vi "Test Gamma jj'.vi"() -> ()   [LabVIEW 2013, in "Zernike Polynome.lvlib"]
doc: "This VI is used to test the calculation of the Zernike polynomial derivative matrix."
uses:
  Zernike Polynome.lvlib
panel:
  out "Array 2":dbl[][](array[numeric])
  out "Array":T1(array[cluster])
  in  "X/Y":bool
  in  "j max (1)":i32=1
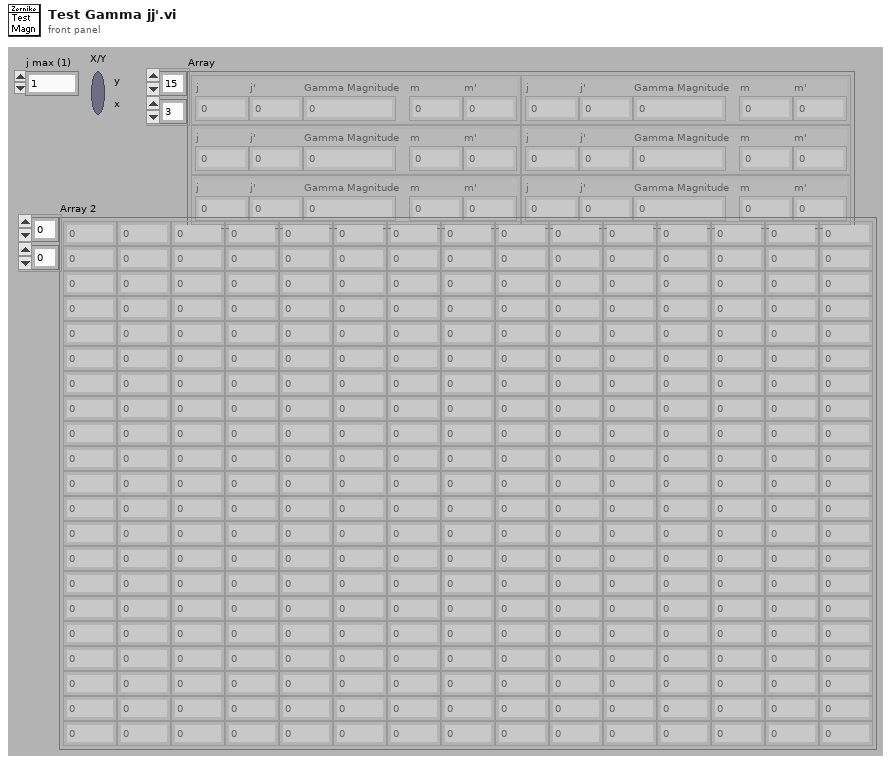
[diagram p1: front panel]
types:
  T1 = cluster{"j":i32, "j'":i32, "Gamma Magnitude":dbl, "m":i32, "m'":i32}[][]
  T2 = cluster{i32, i32, "Gamma Magnitude":dbl, "m":i32, "m'":i32}
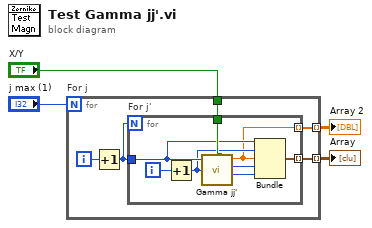
[diagram p0: block diagram]
diagram:
  n1 = for "For j" {
    N: "j max (1)" -> [_]
    tunnel: "X/Y" -> [w8]
    tunnel: [w7] -> w2 mode=indexing
    tunnel: [w5] -> w1 mode=indexing
    i -> [w9]
    n2 = Increment(x=w9) -> (x+1=w6:i32)
    n3 = for "For j'" {
      N: w6 -> [_]
      tunnel: w6 -> [w12]
      tunnel: w8 -> [w16]
      tunnel: [w13] -> w7 mode=indexing
      tunnel: [w10] -> w5 mode=indexing
      i -> [w17]
      n4 = Increment(x=w17) -> (x+1=w11:i32)
      n5 = call "Gamma jj'.vi"("X/Y"=w16, "j' (1)"=w11, "j (1)"=w12) -> ("m'"=w14:i32, "m"=w15:i32, "Gamma Magnitude"=w10:dbl)  [unwired: 1 in, 1 out]
      n6 = Bundle(w12, w11, "Gamma Magnitude"=w10, "m"=w15, "m'"=w14) -> (w13:T2)  [unwired: 1 in]
    }
  }
  "Array" <- w2
  "Array 2" <- w1
